vi "operacionesDeValor.vi"() -> ()   [LabVIEW 2020]
panel:
  in  "U 2":cluster{"Numeric":u8, "Numeric":u8}(slide)={"Numeric"=0, "Numeric"=202} scale=0.0..255.0
  in  "U":u8(slide) scale=0.0..255.0
  in  "Enum":T1(ring)
  out "new picture":picture
  in  "path to JPEG file":path=path "C:/Users/dtrej/Downloads/SVA 06 HISTOGRAMA-20250430T011009Z-001/SVA 06 HISTOGRAMA/1.jpg"
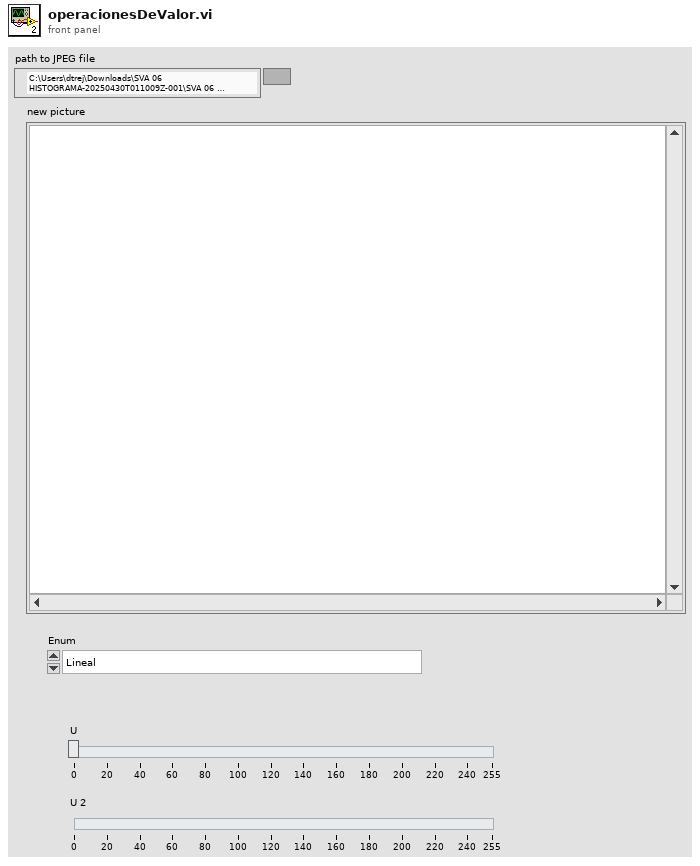
[diagram p1: front panel]
types:
  T1 = enum16{"Lineal", "Invertido", "Umbral", "Umbral invertido", "Umbral doble", "Umbral doble invertido", "Umbral doble en grises", "Umbral doble en grises invertido"}
  T2 = typedef "imagedata.ctl" = cluster{"image type":i32, "image depth":i32, "image":u8[], "mask":u8[], "colors":u32[], "Rectangle":cluster{"left":i16, "top":i16, "right":i16, "bottom":i16}}
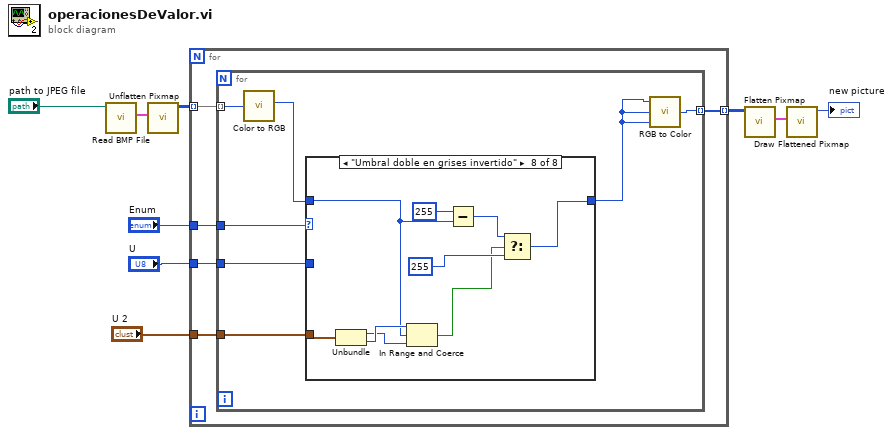
[diagram p0: block diagram]
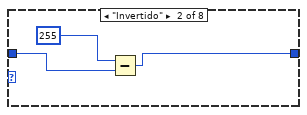
[diagram p3: hidden frame]
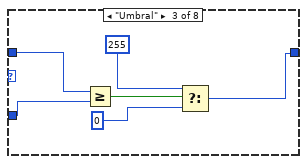
[diagram p4: hidden frame]
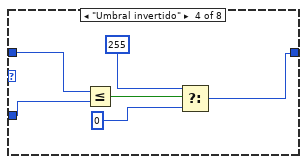
[diagram p5: hidden frame]
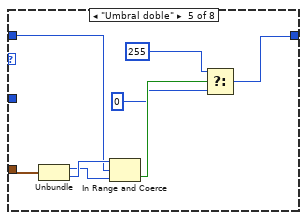
[diagram p6: hidden frame]
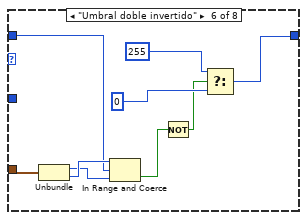
[diagram p7: hidden frame]
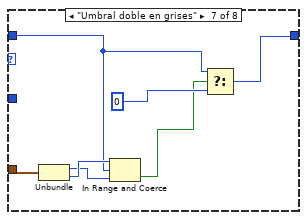
[diagram p8: hidden frame]
diagram:
  n1 = call <vilib>:"Read BMP File.vi"("path to BMP file"="path to JPEG file") -> ("image data"=w8:T2)  [unwired: 8 in, 2 out]
  n2 = call <vilib>:"Unflatten Pixmap.vi"("image data"=w8) -> ("24-bit pixmap"=w7:u32[][])  [unwired: 4 in, 6 out]
  n3 = for {
    tunnel: w7 -> [w14] mode=indexing
    tunnel: [w13] -> w6 mode=indexing
    tunnel: "Enum" -> [w12]
    tunnel: "U" -> [w11]
    tunnel: "U 2" -> [w10]
    n4 = for {
      tunnel: w14 -> [w21] mode=indexing
      tunnel: [w20] -> w13 mode=indexing
      tunnel: w12 -> [w19]
      tunnel: w11 -> [w16]
      tunnel: w10 -> [w15]
      n5 = call <vilib>:"Color to RGB.vi"("Color"=w21) -> ("R"=w17:u8)  [unwired: 3 out]
      n6 = case shown="\"Umbral doble en grises invertido\"" w19 {
        tunnel: w17 -> [w22 w24 w31 w37 w38 w46 w55 w64]
        tunnel: [w22 w23 w26 w32 w39 w49 w57 w66] -> w18
        tunnel: w16 -> [_ _ w30 w36 _ _ _ _]
        tunnel: w15 -> [_ _ _ _ w45 w54 w61 w70]
        frame "Lineal", Default {
        }
        frame "Invertido" {
          n7 = Subtract(x=255, y=w24) -> (x-y=w23:i32)
        }
        frame "Umbral" {
          n8 = Greater Or Equal?(x=w31, y=w30) -> (x >= y?=w29:bool)
          n9 = Select(t=255, s=w29, f=0) -> (s? t:f=w26:i32)
        }
        frame "Umbral invertido" {
          n10 = Less Or Equal?(x=w37, y=w36) -> (x <= y?=w35:bool)
          n11 = Select(t=255, s=w35, f=0) -> (s? t:f=w32:i32)
        }
        frame "Umbral doble" {
          n12 = Unbundle(w45) -> ("Numeric"=w43:u8, "Numeric"=w44:u8)
          n13 = In Range and Coerce(upper limit=w44, x=w38, lower limit=w43) -> (In Range?=w42:bool)  [unwired: 1 out]
          n14 = Select(t=255, s=w42, f=0) -> (s? t:f=w39:i32)
        }
        frame "Umbral doble invertido" {
          n15 = Unbundle(w54) -> ("Numeric"=w52:u8, "Numeric"=w53:u8)
          n16 = In Range and Coerce(upper limit=w53, x=w46, lower limit=w52) -> (In Range?=w47:bool)  [unwired: 1 out]
          n17 = Not(x=w47) -> (.not. x?=w48:bool)
          n18 = Select(t=255, s=w48, f=0) -> (s? t:f=w49:i32)
        }
        frame "Umbral doble en grises" {
          n19 = Unbundle(w61) -> ("Numeric"=w59:u8, "Numeric"=w60:u8)
          n20 = In Range and Coerce(upper limit=w60, x=w55, lower limit=w59) -> (In Range?=w56:bool)  [unwired: 1 out]
          n21 = Select(t=w55, s=w56, f=0) -> (s? t:f=w57:i32)
        }
        frame "Umbral doble en grises invertido" {
          n22 = Unbundle(w70) -> ("Numeric"=w68:u8, "Numeric"=w69:u8)
          n23 = In Range and Coerce(upper limit=w69, x=w64, lower limit=w68) -> (In Range?=w65:bool)  [unwired: 1 out]
          n24 = Subtract(x=u8 255, y=w64) -> (x-y=w62:u8)
          n25 = Select(t=w62, s=w65, f=255) -> (s? t:f=w66:i32)
        }
      }
      n26 = call <vilib>:"RGB to Color.vi"("B"=w18, "G"=w18, "R"=w18) -> ("Color"=w20:u32)
    }
  }
  n27 = call <vilib>:"Flatten Pixmap.vi"("24-bit pixmap"=w6) -> ("image data"=w5:T2)  [unwired: 10 in]
  n28 = call <vilib>:"Draw Flattened Pixmap.vi"("image data"=w5) -> ("new picture"=→"new picture":picture)  [unwired: 8 in]
